vi "Change_Motor_Exp_ID_Address.vi"() -> ()   [LabVIEW 2017]
uses:
  <vilib>/myRIO/Common/Instrument Driver Framework/myRIO v1.0/UART/vis/myRIO v1.0 Close UART.vi
  <vilib>/myRIO/Common/Instrument Driver Framework/Utilities/vis/FPGA Ref Manager.vi
  <vilib>/myRIO/Common/Instrument Driver Framework/myRIO v1.0/myRIO v1.0 Reset FPGA.vi
  <vilib>/myRIO/Common/Instrument Driver Framework/myRIO v1.0/IRQ/vis/myRIO v1.0 IRQ Info FGV.vi
  <vilib>/myRIO/Common/Instrument Driver Framework/myRIO v1.0/IRQ/vis/myRIO v1.0 Timer IRQ Info FGV.vi
  <vilib>/myRIO/Common/Instrument Driver Framework/myRIO v1.0/IRQ/vis/myRIO v1.0 ISR Agent.vi
  <vilib>/myRIO/Instrument Drivers/Utilities/Utilities.lvlib
panel:
  out "error out":errorcluster
  in  "New ID# \n/ I2C Address":u8=1
  in  "Controller ID#  \n(I2C Address)":u8=1 min=1 max=4
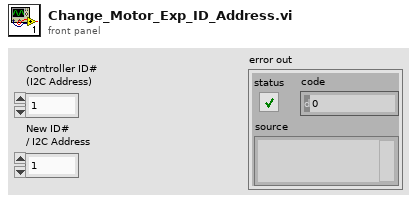
[diagram p1: front panel]
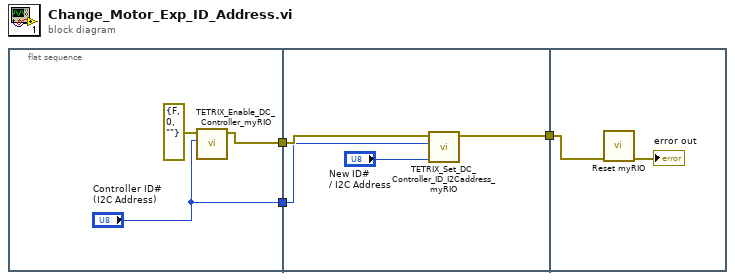
[diagram p0: block diagram]
diagram:
  n1 = flat-sequence {
    tunnel: [w5] -> w3
    tunnel: ["Controller ID#  \n(I2C Address)"] -> w1
    tunnel: w3 -> [w10]
    tunnel: [w9] -> w2
    tunnel: w1 -> [w8]
    tunnel: w2 -> [w12]
    frame #0 {
      n2 = call <vilib>:"TETRIX_Enable_DC_Controller_myRIO.vi"("Controller ID#  (I2C Address)"="Controller ID#  \n(I2C Address)", "Error/Flow In"=errorcluster {"status"=FALSE, "code"=0, "source"=""} ("error constant")) -> ("Error/Flow Out"=w5:errorcluster)  [unwired: 5 in]
    }
    frame #1 {
      n3 = call <vilib>:"TETRIX_Set_DC_Controller_ID_I2Caddress_myRIO.vi"("New ID# / I2C Address"="New ID# \n/ I2C Address", "Current ID#  / I2C Address"=w8, "Error/Flow In"=w10) -> ("Error/Flow Out"=w9:errorcluster)  [unwired: 4 in]
    }
    frame #2 {
      n4 = call <vilib>:"Reset myRIO.vi"("error in (no error)"=w12) -> ("error out"=→"error out":errorcluster)  [unwired: 10 in]
    }
  }
